vi "Record Button Pressed.vi"(8 "error in":errorcluster, 10 "Value":bool, 11 "Signal Name":string) -> (0 "error out":errorcluster)   [LabVIEW 2021, in "UI.lvlib"]
doc: "Record Button Pressed\n_____\nCreated using DQMH Event Scripter 7.0.1.1316."
uses:
  UI.lvlib
  Record Button Pressed Argument--cluster.ctl
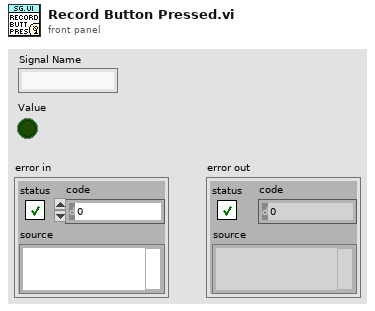
[diagram p1: front panel]
types:
  T1 = typedef "UI.lvlib/Record Button Pressed Argument--cluster.ctl" = cluster{"Value":bool, "Signal Name":string}
  T2 = typedef "UI.lvlib/Broadcast Events--cluster.ctl" = cluster{"Module Did Init":refnum<user-event>, "Status Updated":refnum<user-event>, "Error Reported":refnum<user-event>, "Module Did Stop":refnum<user-event>, "Update Module Execution Status":refnum<user-event>, "Record Button Pressed":refnum<user-event>, "Signal Parameters Changed":refnum<user-event>}
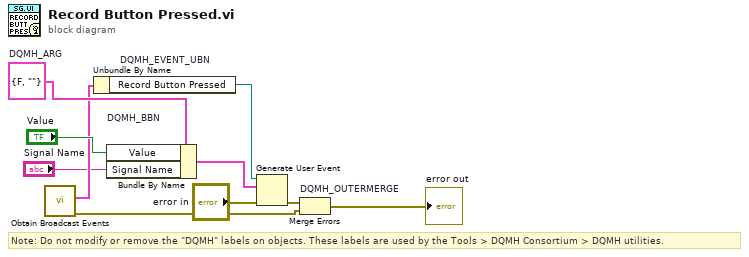
[diagram p0: block diagram]
diagram:
  w5 = T1 {"Value"=FALSE, "Signal Name"=""}  # DQMH_ARG
  # "Note: Do not modify or remove the \"DQMH\" labels on objects. These labels are used by the Tools > DQMH Consortium > DQMH utilities."
  n1 = call "Obtain Broadcast Events.vi"() -> ("error out"=w3:errorcluster, "UI Broadcast Events"=w2:T2)  [unwired: 10 in]
  n2 = Unbundle By Name "DQMH_EVENT_UBN"(w2) -> ("Record Button Pressed"=w7:refnum<user-event>)
  n3 = Bundle By Name "DQMH_BBN"(cluster=w5, "Value"="Value", "Signal Name"="Signal Name") -> (w8:T1)
  n4 = Generate User Event(user event=w7, event data cluster=w8, error in="error in") -> (error out=w6:errorcluster)  [unwired: 1 in, 1 out]
  n5 = Merge Errors "DQMH_OUTERMERGE"(w6, w3) -> (→"error out":errorcluster)
